vi "Collect Actions.vi"(7 "Round":u32, 9 "Teams In":refnum<class "Team.lvclass">[](array[class]), 11 "Map in":refnum<class "Map.lvclass">) -> (1 "Teams":refnum<class "Team.lvclass">[](array[class]), 3 "Map out":refnum<class "Map.lvclass">)   [LabVIEW 2020, in "SquareBattle.lvlib" / "Map.lvclass"]
uses:
  Map.lvclass
  Team/Team.lvclass
  Map.lvclass/Map.ctl
  Position.ctl
  Square/Square.lvclass/Square.ctl
  Run Result.ctl
  Action.ctl
  Direction.ctl
  Square/Square.lvclass
  Direction Position Offsets.vi
  SquareBattle.lvlib
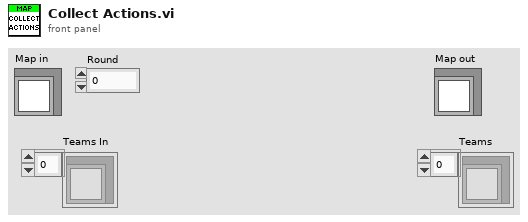
[diagram p1: front panel]
types:
  T1 = typedef "SquareBattle.lvlib/Position.ctl" = cluster{"Row":i32, "Col":i32}
  T2 = typedef "SquareBattle.lvlib/Run Result.ctl" = cluster{"Action":T3, "Direction":T4, "Replication":refnum<class "Square.lvclass">}
  T3 = typedef "SquareBattle.lvlib/Action.ctl" = enum16{"Wait", "Move", "Attack", "Replicate"}
  T4 = typedef "SquareBattle.lvlib/Direction.ctl" = enum16{"NW", "N", "NE", "E", "SE", "S", "SW", "W"}
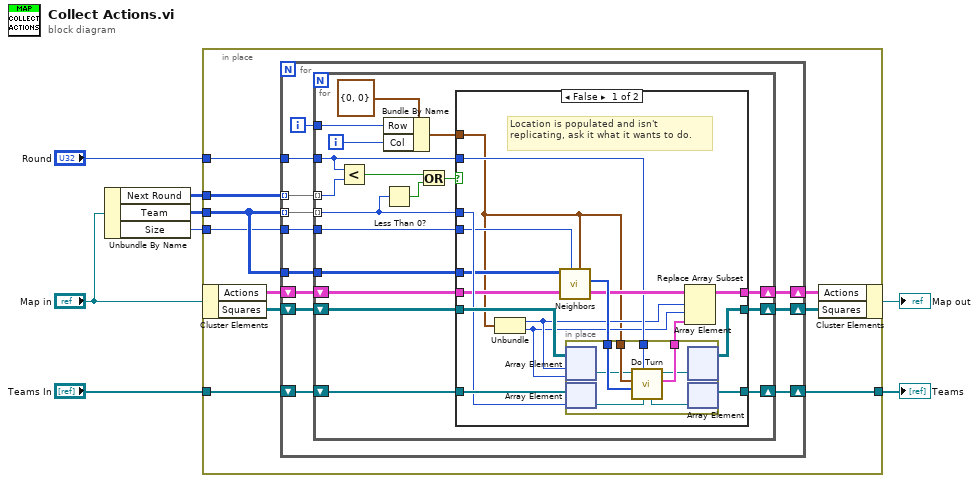
[diagram p0: block diagram]
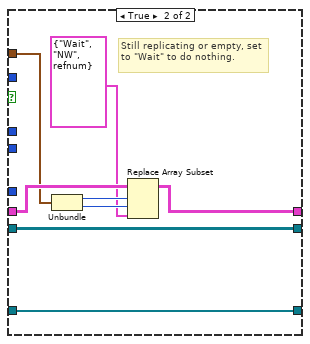
[diagram p2: hidden frame]
diagram:
  n1 = Unbundle By Name("Map in") -> ("Next Round"=w8:u32[][], "Team"=w7:i32[][], "Size"=w1:i32)
  n2 = in-place {
    in-place-border: "Round" -> [w15]
    in-place-border: "Teams In" -> [w18]
    in-place-border: [w14] -> w2
    in-place-border: w8 -> [w13]
    in-place-border: w7 -> [w10]
    in-place-border: w1 -> [w9]
    n3 = in-place-cluster #1("Map in") -> ("Actions"=w12:T2[][], "Squares"=w17:refnum<class "Square.lvclass">[][])
    n4 = for {
      shift-right: [w29] -> w14
      shift-left: w18 -> [w30]
      shift-right: [w27] -> w16
      shift-left: w17 -> [w28]
      shift-right: [w23] -> w11
      shift-left: w12 -> [w26]
      tunnel: w15 -> [w24]
      tunnel: w13 -> [w22] mode=indexing
      tunnel: w10 -> [w21] mode=indexing
      tunnel: w10 -> [w20]
      tunnel: w9 -> [w19]
      i -> [w25]
      n5 = for {
        shift-right: [w43] -> w29
        shift-left: w30 -> [w48]
        shift-right: [w44] -> w27
        shift-left: w28 -> [w47]
        shift-right: [w45] -> w23
        shift-left: w26 -> [w46]
        tunnel: w25 -> [w39]
        tunnel: w24 -> [w33]
        tunnel: w22 -> [w34] mode=indexing
        tunnel: w21 -> [w36] mode=indexing
        tunnel: w20 -> [w35]
        tunnel: w19 -> [w31]
        i -> [w38]
        n6 = Less?(x=w33, y=w34) -> (x < y?=w32:bool)
        n7 = Bundle By Name(cluster=T1 {"Row"=0, "Col"=0} ("Position"), "Row"=w39, "Col"=w38) -> (w37:T1)
        n8 = Less Than 0?(x=w36) -> (x < 0?=w42:bool)
        n9 = Or(x=w32, y=w42) -> (x .or. y?=w41:bool)
        n10 = case shown="False" w41 {
          tunnel: w48 -> [w62 w78]
          tunnel: w47 -> [w63 w79]
          tunnel: w46 -> [w58 w77]
          tunnel: [w56 w72] -> w45
          tunnel: [w55 w79] -> w44
          tunnel: [w59 w78] -> w43
          tunnel: w36 -> [w61 _]
          tunnel: w37 -> [w49 w74]
          tunnel: w35 -> [w54 _]
          tunnel: w33 -> [w53 _]
          tunnel: w31 -> [w50 _]
          frame False {
            # "Location is populated and isn't replicating, ask it what it wants to do."
            n11 = Unbundle(w49) -> ("Row"=w52:i32, "Col"=w51:i32)
            n12 = call "Neighbors.vi"("Position"=w49, "Board Size"=w50, "Team In"=w54) -> ("Neighbors"=w60:i32[])  [unwired: 7 in, 1 out]
            n13 = in-place {
              in-place-border: w53 -> [w71]
              in-place-border: w49 -> [w70]
              in-place-border: w60 -> [w69]
              in-place-border: [w66] -> w57
              n14 = in-place-array #2(w63, w52, w51) -> (w65:refnum<class "Square.lvclass">)
              n15 = in-place-array #3(w62, w61) -> (w68:refnum<class "Team.lvclass">)
              n16 = call "Do Turn.vi"("Team in"=w68, "Round Number"=w71, "Neighbors"=w69, "Position"=w70, "Square in"=w65) -> ("Run Result"=w66:T2, "Square out"=w64:refnum<class "Square.lvclass">, "Team out"=w67:refnum<class "Team.lvclass">)  [unwired: 4 in]
              n17 = in-place-array #2(w64) -> (w55:refnum<class "Square.lvclass">[][])  [unwired: 2 out]
              n18 = in-place-array #3(w67) -> (w59:refnum<class "Team.lvclass">[])  [unwired: 1 out]
            }
            n19 = Replace Array Subset(array=w58, new element=w57, index (row)=w52, index (col)=w51) -> (w56:T2[][])
          }
          frame True {
            # "Still replicating or empty, set to \"Wait\" to do nothing."
            n20 = Unbundle(w74) -> ("Row"=w76:i32, "Col"=w75:i32)
            n21 = Replace Array Subset(array=w77, new element=T2 {"Action"=enum."Wait", "Direction"=enum."NW", "Replication"=refnum} ("new element/subarray"), index (row)=w76, index (col)=w75) -> (w72:T2[][])
          }
        }
      }
    }
    n22 = in-place-cluster #1("Actions"=w11, "Squares"=w16) -> (→"Map out":refnum<class "Map.lvclass">)
  }
  "Teams" <- w2
